vi "Controller Timing Initialize.vi"(10 "Controller - User Input":T2, 11 "Controller Select":T1(ring)=enum."100hz/100hz" caption="Enum") -> (0 "error out":errorcluster, 3 "IMU_sample_rate":i32)   [LabVIEW 2014]
uses:
  Start.vi
panel:
  in  "error in":errorcluster
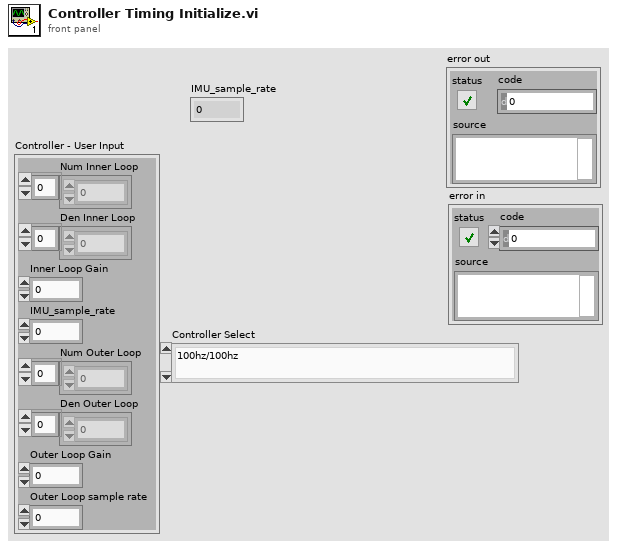
[diagram p1: front panel]
types:
  T1 = enum16{"100hz/50hz", "100hz/100hz", "200hz/200hz", "200hz/20hz", "User Defined"}
  T2 = cluster{"Num Inner Loop":dbl[], "Den Inner Loop":dbl[], "Inner Loop Gain":dbl, "IMU_sample_rate":i32, "Num Outer Loop":dbl[], "Den Outer Loop":dbl[], "Outer Loop Gain":dbl, "Outer Loop sample rate":dbl}
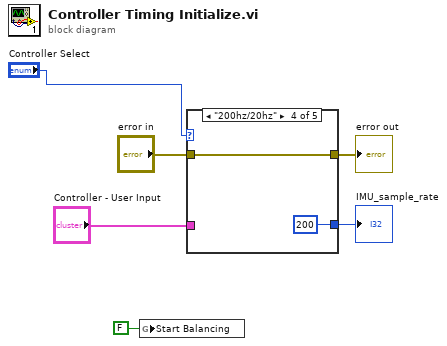
[diagram p0: block diagram]
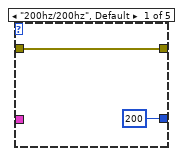
[diagram p2: hidden frame]
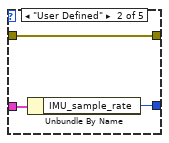
[diagram p3: hidden frame]
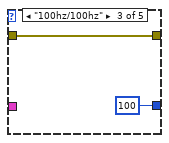
[diagram p4: hidden frame]
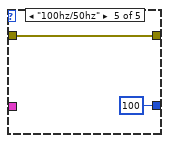
[diagram p5: hidden frame]
diagram:
  n1 = global write "Start.vi" "Start Balancing"(FALSE ("Start Balancing")) -> ()
  n2 = case shown="\"200hz/20hz\"" "Controller Select" {
    tunnel: [200 w10 100 ("IMU_sample_rate") 200 100 ("IMU_sample_rate")] -> w5
    tunnel: "Controller - User Input" -> [_ w11 _ _ _]
    tunnel: [w7 w9 w12 w14 w17] -> w4
    tunnel: "error in" -> [w7 w9 w12 w14 w17]
    frame "200hz/200hz", Default {
    }
    frame "User Defined" {
      n3 = Unbundle By Name(w11) -> ("IMU_sample_rate"=w10:i32)
    }
    frame "100hz/100hz" {
    }
    frame "200hz/20hz" {
    }
    frame "100hz/50hz" {
    }
  }
  "IMU_sample_rate" <- w5
  "error out" <- w4
